vi "Engine Start Control Handler.vi"(6 "Engine Shutdown Delay (ms)":u32=20000, 7 "Engine Start Control":T1 scale=0.0..2.0, 8 "error in (no error)":errorcluster, 9 "Engine Start Delay (ms)":u32=8000, 10 "RUN Ref":refnum<vi>, 11 "Engine Start Control Ref":refnum<vi>) -> (0 "error out":errorcluster, 2 "Inlet Door":bool)   [LabVIEW 2018]
uses:
  Public Controls/Engine Start Control.ctl
  cRIO RT Comms/Private Controls/Stream Data.ctl
  50cbc6c0-c243-4a21-83be-8cf143a89abc.vi
  490cb36f-2560-4867-b935-1e557128a452.vi
  cRIO RT Comms/cRIO RT Comms.lvlib
panel:
  out "RUN 2":bool=TRUE caption="OPEN"
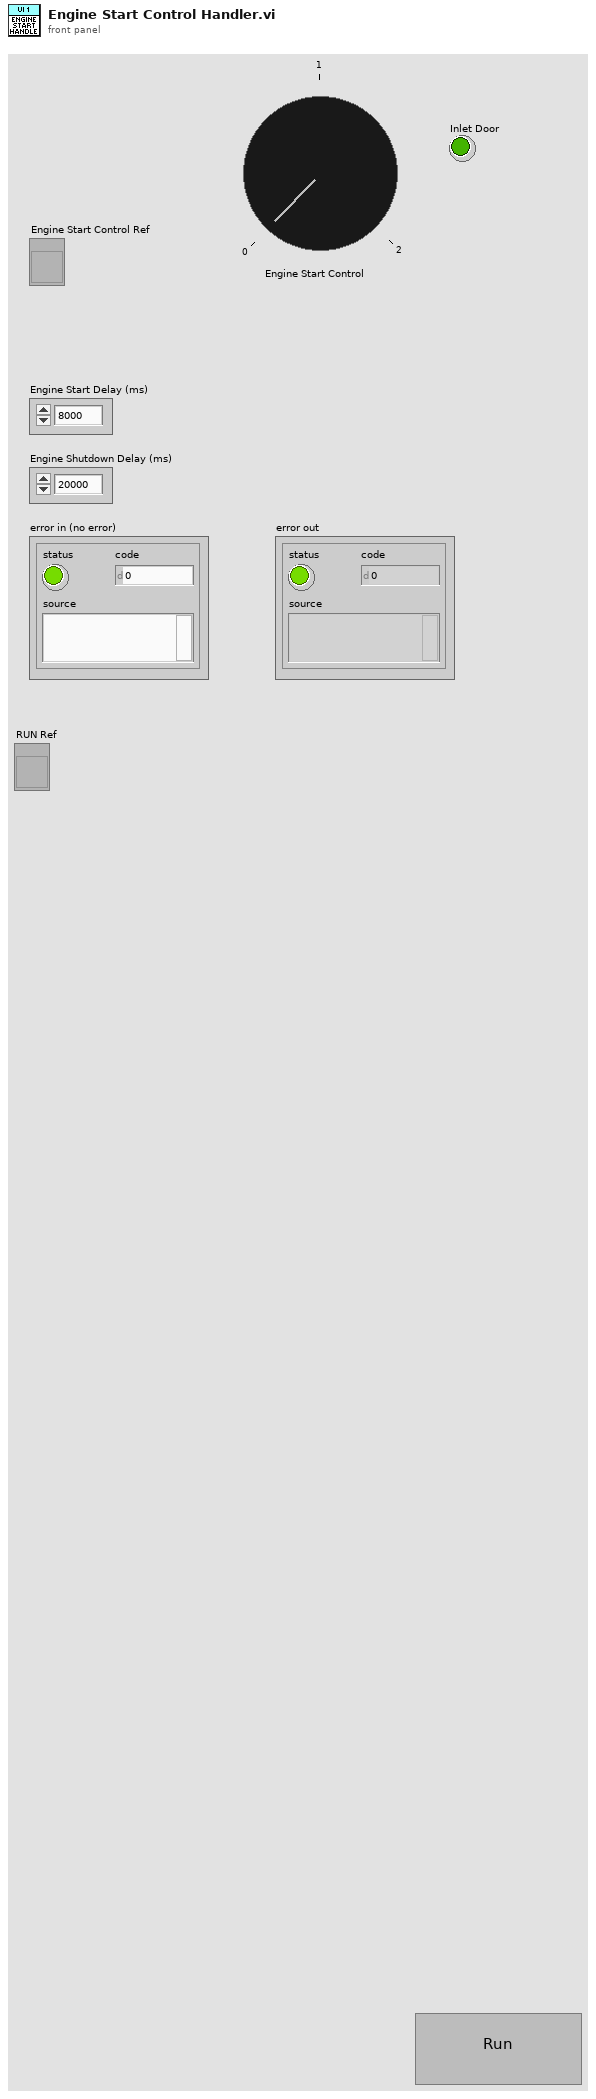
[diagram p1: front panel]
types:
  T1 = typedef "Engine Start Control.ctl" = u8
  T2 = typedef "cRIO RT Comms.lvlib/Stream Data.ctl" = cluster{"Action":string, "Data":variant}
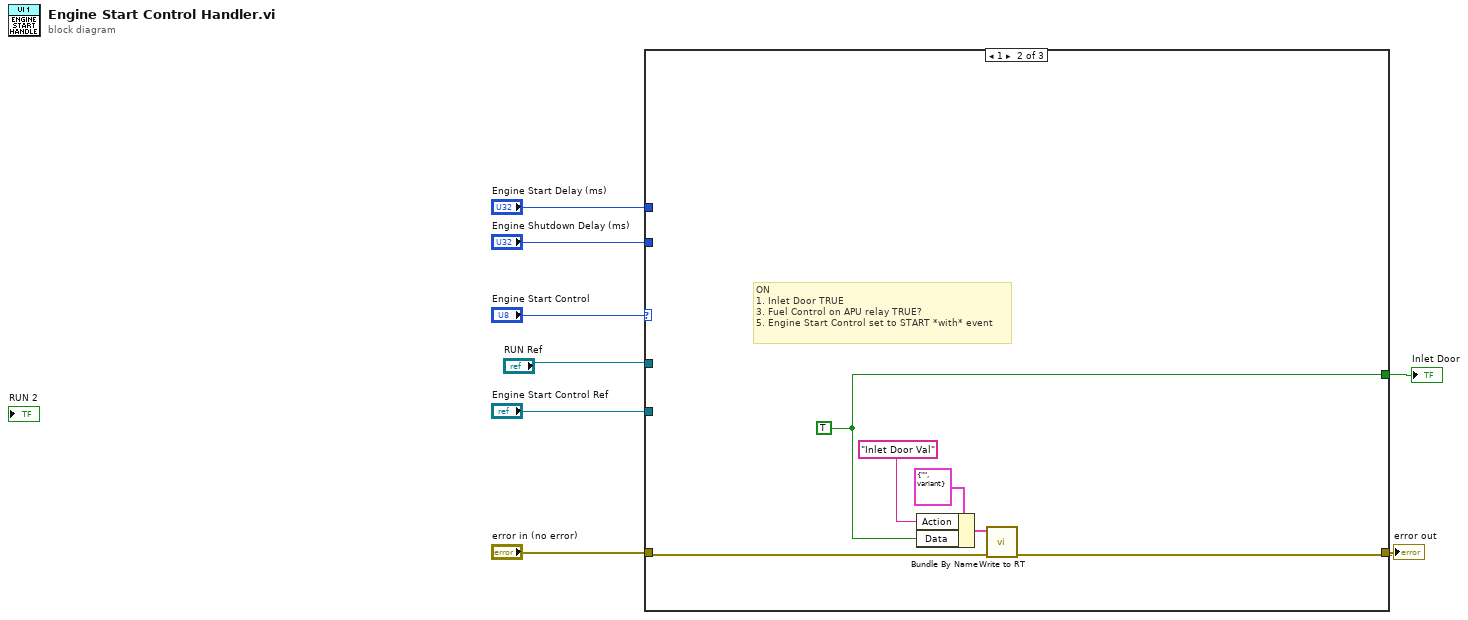
[diagram p0: block diagram]
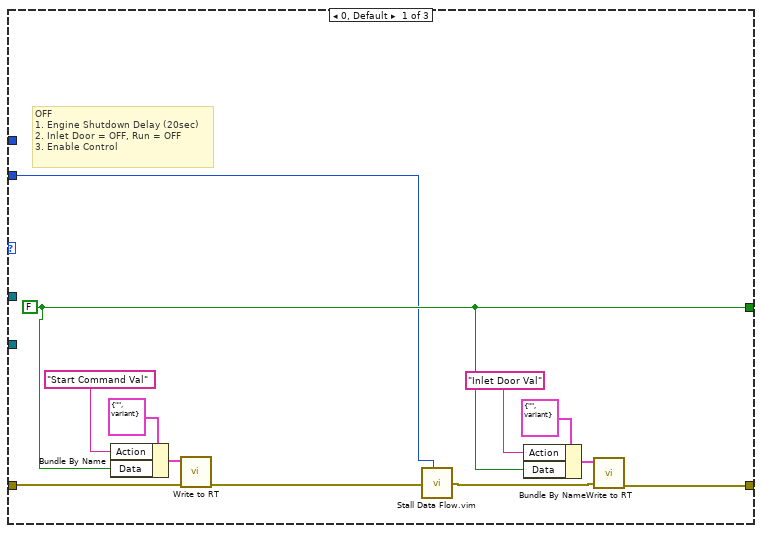
[diagram p2: hidden frame]
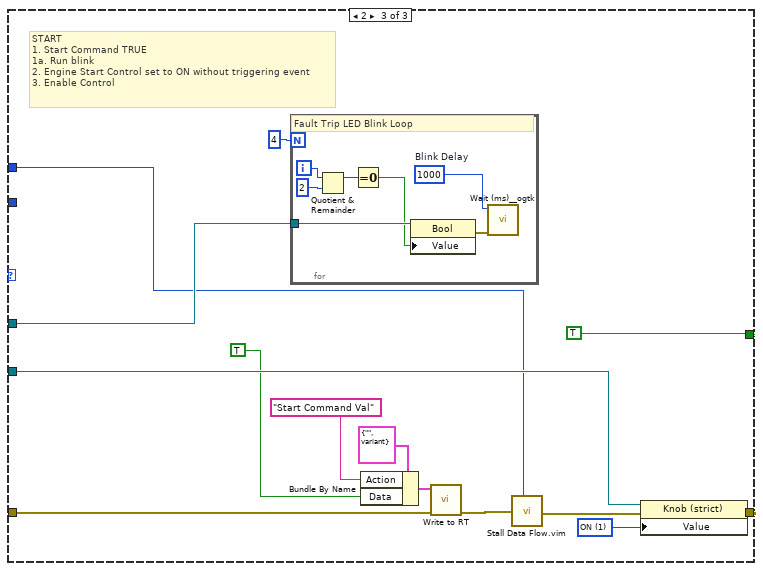
[diagram p3: hidden frame]
diagram:
  n1 = case shown="1" "Engine Start Control" {
    tunnel: [w12 w21 w38] -> w2
    tunnel: "error in (no error)" -> [w14 w22 w40]
    tunnel: "Engine Start Control Ref" -> [_ _ w37]
    tunnel: "RUN Ref" -> [_ _ w39]
    tunnel: [w13 w23 TRUE] -> w5
    tunnel: "Engine Shutdown Delay (ms)" -> [w11 _ _]
    tunnel: "Engine Start Delay (ms)" -> [_ _ w36]
    frame 0, Default {
      w13 = FALSE
      # "OFF\n1. Engine Shutdown Delay (20sec)\n2. Inlet Door = OFF, Run = OFF\n3. Enable Control"
      n2 = Bundle By Name(cluster=T2 {"Action"="", "Data"=variant} ("Data to Write"), "Action"="Start Command Val", "Data"=w13) -> (w16:T2)
      n3 = call "Write to RT.vi"("error in (no error)"=w14, "Data to Write"=w16) -> ("error out"=w9:errorcluster)  [unwired: 9 in]
      n4 = call "Stall Data Flow.vim"("value in"=w9, "milliseconds to wait"=w11) -> ("value out"=w10:errorcluster)  [unwired: 1 out]
      n5 = Bundle By Name(cluster=T2 {"Action"="", "Data"=variant} ("Data to Write"), "Action"="Inlet Door Val", "Data"=w13) -> (w19:T2)
      n6 = call "Write to RT.vi"("error in (no error)"=w10, "Data to Write"=w19) -> ("error out"=w12:errorcluster)  [unwired: 9 in]
    }
    frame 1 {
      w23 = TRUE
      # "ON\n1. Inlet Door TRUE\n3. Fuel Control on APU relay TRUE?\n5. Engine Start Control set to START *with* event"
      n7 = Bundle By Name(cluster=T2 {"Action"="", "Data"=variant} ("Data to Write"), "Action"="Inlet Door Val", "Data"=w23) -> (w25:T2)
      n8 = call "Write to RT.vi"("error in (no error)"=w22, "Data to Write"=w25) -> ("error out"=w21:errorcluster)  [unwired: 9 in]
    }
    frame 2 {
      w27 = T1 1 items=["OFF", "ON", "START"] ("Engine Start Control")
      # "START\n1. Start Command TRUE\n1a. Run blink\n2. Engine Start Control set to ON without triggering event\n3. Enable Control"
      n9 = for {
        N: 4 -> [_]
        tunnel: w39 -> [w42]
        i -> [w47]
        w43 = u32 1000  # Blink Delay
        # "Fault Trip LED Blink Loop"
        n10 = Quotient & Remainder(x=w47, y=2) -> (x-y*floor(x/y)=w45:i32)  [unwired: 1 out]
        n11 = Equal To 0?(x=w45) -> (x = 0?=w41:bool)
        n12 = property on="Property Node" class="Bool"(reference=w42, "Value"=w41) -> (error out=w44:errorcluster)  [unwired: 1 in, 1 out]
        n13 = call <userlib>:"Wait (ms)__ogtk.vi"("error in (no error)"=w44, "milliseconds to wait"=w43) -> ()  [unwired: 8 in, 2 out]
      }
      n14 = Bundle By Name(cluster=T2 {"Action"="", "Data"=variant} ("Data to Write"), "Action"="Start Command Val", "Data"=TRUE) -> (w32:T2)
      n15 = call "Write to RT.vi"("error in (no error)"=w40, "Data to Write"=w32) -> ("error out"=w30:errorcluster)  [unwired: 9 in]
      n16 = call "Stall Data Flow.vim"("value in"=w30, "milliseconds to wait"=w36) -> ("value out"=w34:errorcluster)  [unwired: 1 out]
      n17 = property class="Knob (strict)"(reference=w37, error in=w34, "Value"=w27) -> (error out=w38:errorcluster)  [unwired: 1 out]
    }
  }
  "error out" <- w2
  "Inlet Door" <- w5
